vi "Check etc-hosts.vi"(8 "error in":errorcluster, 11 "address":refnum<class "Hostname Network Address.lvclass">) -> (0 "error out":errorcluster, 3 "resolved addresses":refnum<class "Generic Network Address.lvclass">[](array[class]))   [LabVIEW 2020, in "NI_WFCN.lvlib" / "Hostname Network Address.lvclass"]
doc: "Look up the specified hostname in /etc/hosts (or its equivalent). Multiple addresses may be returned, if resolution succeeded through multiple protocols. If no results were found, returns an empty array."
uses:
  <vilib>/net/WFCN/Addressing/Hostname Network Address/Hostname Network Address.lvclass
  e:/builds/penguin/labview/branches/2020/dev/dist/vi.lib/net/WFCN/Addressing/Generic Network Address/Generic Network Address.lvclass
  <vilib>/net/WFCN/Addressing/Generic Network Address/Generic Network Address.lvclass
  <vilib>/net/WFCN/Addressing/Hostname Network Address/Hostname Network Address.lvclass/Hostname Network Address.ctl
  <vilib>/net/WFCN/Addressing/IPv4 Network Address/IPv4 Network Address.lvclass/IPv4 Network Address.ctl
  <vilib>/net/WFCN/Addressing/Generic Network Address/Generic Network Address.lvclass/Generic Network Address.ctl
  <vilib>/net/WFCN/Addressing/Generic Network Address/Parse.vi
  <vilib>/Utility/error.llb/Clear Errors.vi
  <vilib>/net/WFCN/Addressing/Hostname Network Address/Create from string.vi
  <vilib>/net/WFCN/Utility/Is IPv4 address.vi
  <vilib>/net/WFCN/Addressing/IPv4 Network Address/Create from U32.vi
  <vilib>/net/WFCN/Addressing/Generic Network Address/Create for unparsable.vi
  <vilib>/net/WFCN/Utility/Is hostname mDNS.vi
  <vilib>/dlg_ctls.llb/Space Constant.vi
  <vilib>/net/WFCN/Addressing/IPv4 Network Address/IPv4 Network Address.lvclass
  <vilib>/net/WFCN/Addressing/mDNS Hostname Network Address/mDNS Hostname Network Address.lvclass
  e:/builds/penguin/labview/branches/2020/dev/dist/vi.lib/net/WFCN/Addressing/Hostname Network Address/Hostname Network Address.lvclass
  <vilib>/Utility/error.llb/Error Cluster From Error Code.vi
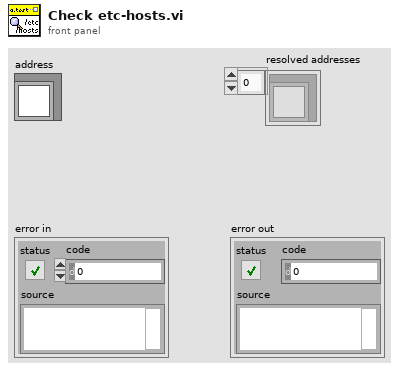
[diagram p1: front panel]
types:
  T1 = enum16{"big-endian, network order", "native, host order", "little-endian"}
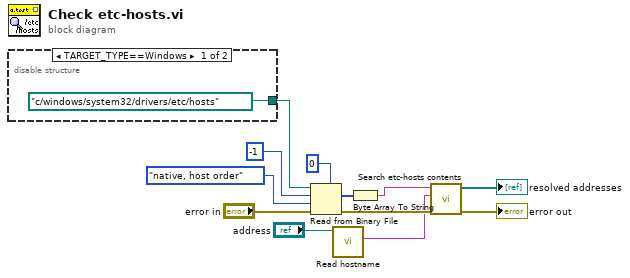
[diagram p0: block diagram]
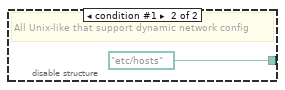
[diagram p2: hidden frame]
diagram:
  n1 = disable-structure shown="TARGET_TYPE==Windows" {
    disable-tunnel: [path "c:/windows/system32/drivers/etc/hosts" path "/etc/hosts"] -> w11
    frame condition #0 (active) {
    }
    frame condition #1 {
      # "All Unix-like that support dynamic network config"
    }
  }
  n2 = Read from Binary File(5:u8 0, 8:"error in", 9:T1."native, host order" ("byte order (0:big-endian, network order)"), 10:-1 ("count (1)"), 11:w11) -> (0:w6:errorcluster, 2:w5:u8[])  [unwired: 1 in, 2 out]
  n3 = call <vilib>:"Read hostname.vi"("address"="address") -> ("hostname"=w2:string)  [unwired: 9 in, 1 out]
  n4 = Byte Array To String(unsigned byte array=w5) -> (string=w4:string)
  n5 = call <vilib>:"Search etc-hosts contents.vi"("error in (no error)"=w6, "hostname"=w2, "/etc/hosts contents"=w4) -> ("error out"=→"error out":errorcluster, "addresses"=→"resolved addresses":refnum<class "Generic Network Address.lvclass">[])  [unwired: 7 in]
